vi "7HP_Convert serial string to Eng vals.vi"(0 "Serial buffer string (excluding FrameChar)":string) -> (9 "All vals":sgl[](array[numeric]), 12 "Pressures":sgl[][](graph), 13 "Gyration vector (deg / s)":sgl[](array[numeric]), 14 "External thermistor temperature (deg C)":sgl, 15 "Atmospheric pressure (mbar)":sgl, 17 "Env. sensor die temperature (deg C)":sgl, 18 "Relative humidity (%)":sgl, 19 "Acceleration vector (g)":sgl[](array[numeric]))   [LabVIEW 2021]
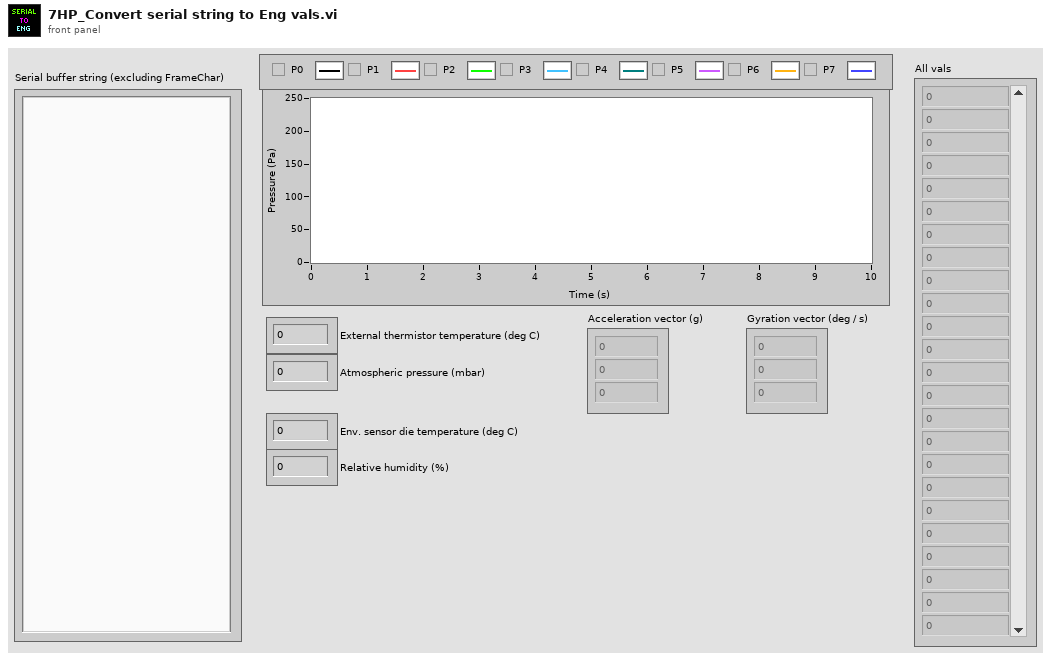
[diagram p1: front panel]
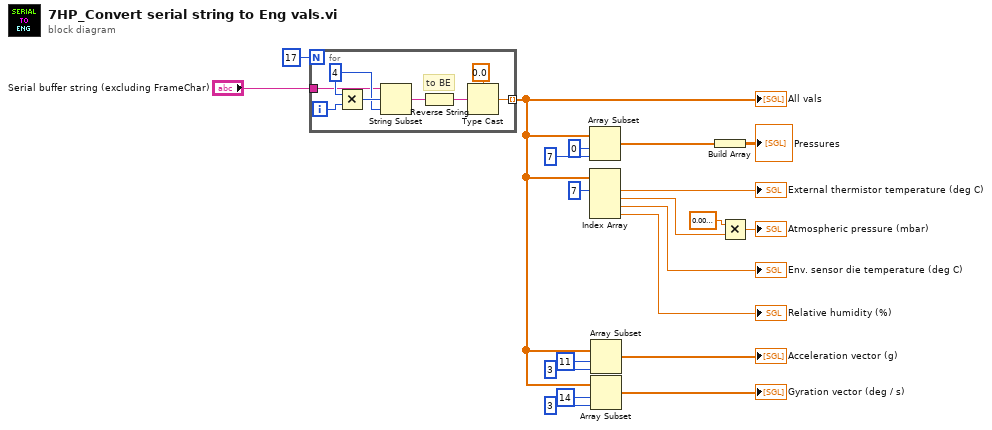
[diagram p0: block diagram]
diagram:
  n1 = for {
    N: 17 -> [_]
    tunnel: [w22] -> w1 mode=indexing
    tunnel: "Serial buffer string (excluding FrameChar)" -> [w21]
    i -> [w28]
    w26 = 4 ("x")
    # "to BE"
    n2 = Multiply(x=w26, y=w28) -> (x*y=w27:i32)
    n3 = String Subset(string=w21, offset (0)=w27, length (rest)=w26) -> (substring=w25:string)
    n4 = Reverse String(1:w25) -> (0:w24:string)
    n5 = Type Cast(type=sgl 0.0 ("byte count"), x=w24) -> (*(type *) &x=w22:sgl)
  }
  "All vals" <- w1
  n6 = Array Subset(array=w1, index=0, length=7) -> (w7:sgl[])
  n7 = Index Array(array=w1, index #1=7 ("index")) -> (element #1=→"External thermistor temperature (deg C)":sgl, element #2=w4:sgl, element #3=→"Env. sensor die temperature (deg C)":sgl, element #4=→"Relative humidity (%)":sgl)  [unwired: 3 in]
  n8 = Array Subset(array=w1, index=11, length=3) -> (→"Acceleration vector (g)":sgl[])
  n9 = Array Subset(array=w1, index=14, length=3) -> (→"Gyration vector (deg / s)":sgl[])
  n10 = Build Array(w7) -> (→"Pressures":sgl[][])
  n11 = Multiply(x=sgl 0.01, y=w4) -> (x*y=→"Atmospheric pressure (mbar)":sgl)
